vi "Query Float.vi"(8 "error in (no error)":errorcluster, 10 "write buffer":string, 11 "VISA resource name In":refnum<visa-resource-name>) -> (0 "error out":errorcluster, 2 "float":dbl, 3 "VISA resource name out":refnum<visa-resource-name>)   [LabVIEW 2023, in "Newport 1830-C.lvlib"]
doc: "Reads a float from the output buffer of the instrument."
uses:
  Newport 1830-C.lvlib
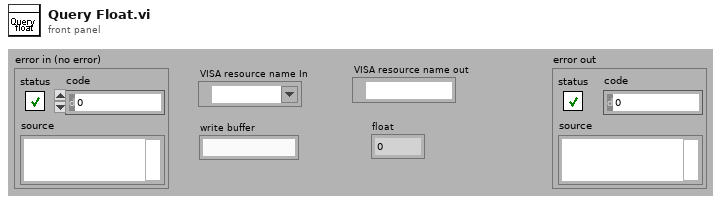
[diagram p1: front panel]
types:
  T1 = typedef "Semaphore RefNum" = refnum<k1>
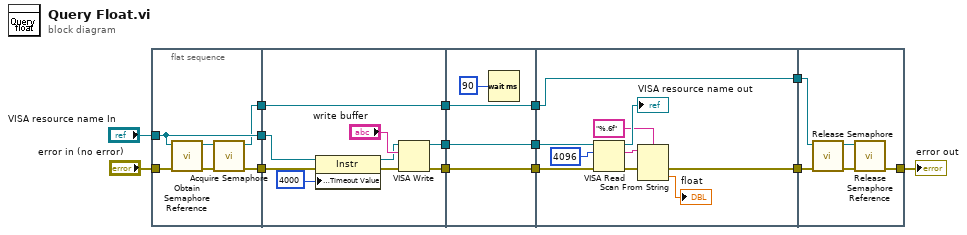
[diagram p0: block diagram]
diagram:
  n1 = flat-sequence {
    tunnel: "VISA resource name In" -> [w17]
    tunnel: "error in (no error)" -> [w20]
    tunnel: [w17] -> w12
    tunnel: [w16] -> w11
    tunnel: [w15] -> w1
    tunnel: w12 -> [w25]
    tunnel: w11 -> [w24]
    tunnel: [w28] -> w9
    tunnel: [w27] -> w7
    tunnel: [w26] -> w2
    tunnel: w1 -> [w26]
    tunnel: [w32] -> w10
    tunnel: w9 -> [w32]
    tunnel: [w31] -> w8
    tunnel: w7 -> [w31]
    tunnel: [w30] -> w3
    tunnel: w2 -> [w30]
    tunnel: w10 -> [w37]
    tunnel: w8 -> [w36]
    tunnel: [w35] -> w6
    tunnel: [w34] -> w4
    tunnel: w3 -> [w34]
    tunnel: w6 -> [w48]
    tunnel: [w46] -> w5
    tunnel: w4 -> [w45]
    frame #0 {
      n2 = call <vilib>:"Obtain Semaphore Reference.vi"("error in (no error)"=w20, "name (unnamed)"=w17) -> ("error out"=w19:errorcluster, "semaphore"=w18:T1)  [unwired: 3 in, 1 out]
      n3 = call <vilib>:"Acquire Semaphore.vi"("error in (no error)"=w19, "semaphore"=w18) -> ("error out"=w16:errorcluster, "semaphore out"=w15:T1)  [unwired: 3 in, 1 out]
    }
    frame #1 {
      n4 = property class="Instr"(reference=w25, error in=w24, "General Settings:Timeout Value"=u32 4000) -> (reference out=w23:refnum<visa-resource-name>, error out=w22:errorcluster)
      n5 = VISA Write(VISA resource name=w23, write buffer="write buffer", error in (no error)=w22) -> (VISA resource name out=w28:refnum<visa-resource-name>, error out=w27:errorcluster)  [unwired: 1 out]
    }
    frame #2 {
      n6 = Wait (ms)(milliseconds to wait=u32 90) -> ()  [unwired: 1 out]
    }
    frame #3 {
      n7 = VISA Read(VISA resource name=w37, byte count=u32 4096, error in (no error)=w36) -> (VISA resource name out=→"VISA resource name out":refnum<visa-resource-name>, read buffer=w40:string, error out=w41:errorcluster)  [unwired: 1 out]
      n8 = Scan From String(format string="%.6f", input string=w40, error in=w41) -> (error out=w35:errorcluster, output 1=→"float":dbl)  [unwired: 2 in, 2 out]
    }
    frame #4 {
      n9 = call <vilib>:"Release Semaphore.vi"("error in (no error)"=w48, "semaphore"=w45) -> ("error out"=w47:errorcluster, "semaphore out"=w44:T1)  [unwired: 4 in]
      n10 = call <vilib>:"Release Semaphore Reference.vi"("error in (no error)"=w47, "semaphore"=w44) -> ("error out"=w46:errorcluster)  [unwired: 8 in, 1 out]
    }
  }
  "error out" <- w5
